vi "FPGA Counts.vi"(0 "saveData":bool, 2 "runs":i32, 5 "fpgaCommand":u8, 7 "fileName":string, 11 "error in (no error)":errorcluster) -> (4 "function return":i32, 10 "length out":i32, 12 "data":i64[](array[numeric]), 13 "stats":i64[](array[numeric]), 15 "error out":errorcluster)   [LabVIEW 2012]
uses:
  x64/Stats.lvlib
  x86/Stats32.lvlib
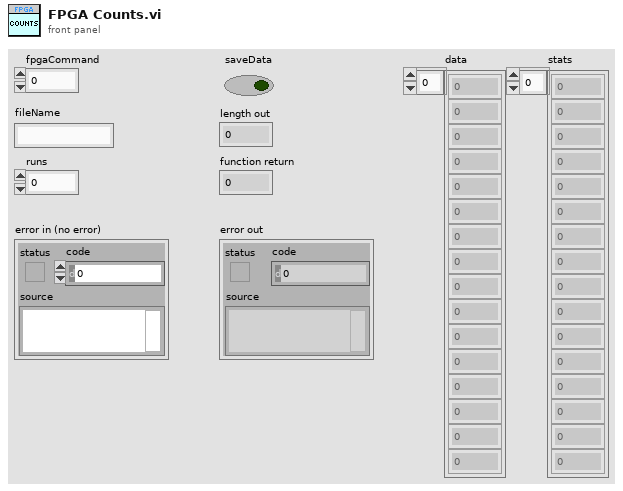
[diagram p1: front panel]
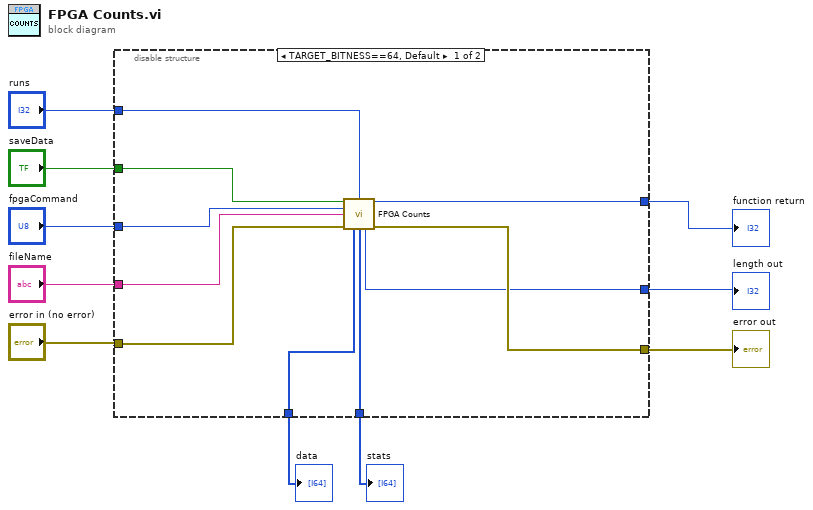
[diagram p0: block diagram]
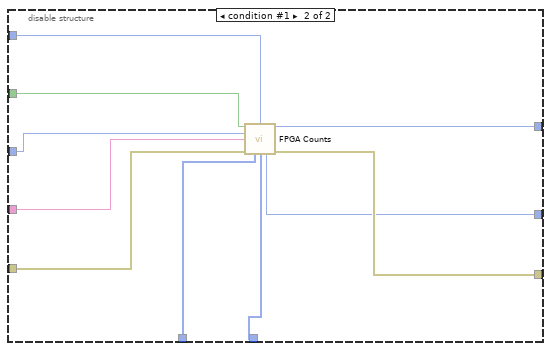
[diagram p2: hidden frame]
diagram:
  n1 = disable-structure shown="TARGET_BITNESS==64, Default" {
    disable-tunnel: "error in (no error)" -> [w20 w28]
    disable-tunnel: [w19 w30] -> w9
    disable-tunnel: [w18 w29] -> w8
    disable-tunnel: "saveData" -> [w17 w25]
    disable-tunnel: "fpgaCommand" -> [w16 w26]
    disable-tunnel: "fileName" -> [w15 w27]
    disable-tunnel: "runs" -> [w14 w24]
    disable-tunnel: [w11 w21] -> w3
    disable-tunnel: [w13 w23] -> w2
    disable-tunnel: [w12 w22] -> w1
    frame condition #0 (active) {
      n2 = call "FPGA Counts.vi"("saveData"=w17, "runs"=w14, "fpgaCommand"=w16, "fileName"=w15, "error in (no error)"=w20) -> ("function return"=w18:i32, "data"=w13:i64[], "stats"=w12:i64[], "length"=w11:i32, "error out"=w19:errorcluster)  [unwired: 6 in]
    }
    frame condition #1 {
      n3 = call "FPGA Counts.vi"("saveData"=w25, "runs"=w24, "fpgaCommand"=w26, "fileName"=w27, "error in (no error)"=w28) -> ("function return"=w29:i32, "Data"=w23:u64[], "Stats"=w22:i64[], "length out"=w21:i32, "error out"=w30:errorcluster)  [unwired: 5 in, 1 out]
    }
  }
  "error out" <- w9
  "function return" <- w8
  "length out" <- w3
  "data" <- w2
  "stats" <- w1
